vi "Request Data From Flash.vi"() -> (3 "DSM Message":string)   [LabVIEW 2014, in "GEA2_Toolkit.lvlib"]
uses:
  Labview GEA2 Toolkit v2.1/library/GEA2_Toolkit.lvlib
  Custom Pallet Controls/Forward.ctl
panel:
  in  "Number of Bytes (up to 16)":u16
  in  "Starting Index in Record (0-255)":u16
  in  "Record Number (0-Max Record Number)":u16
  out "Description":string="Set Currents"
  in  "Complete":T1
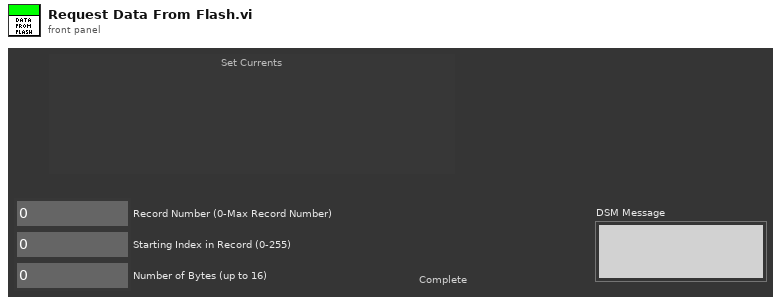
[diagram p1: front panel]
types:
  T1 = typedef "GEA2_Toolkit.lvlib/Forward.ctl" = bool
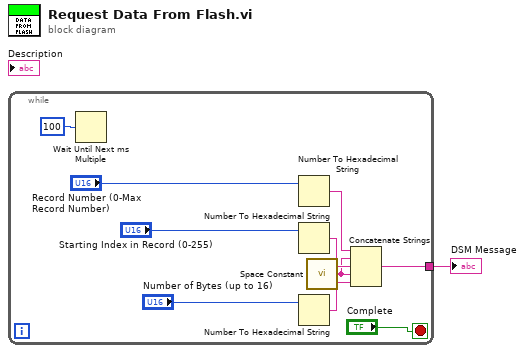
[diagram p0: block diagram]
diagram:
  n1 = while {
    tunnel: [w6] -> w1
    stop <- "Complete" stop-if-true
    n2 = Wait Until Next ms Multiple(millisecond multiple=u32 100) -> ()  [unwired: 1 out]
    n3 = Number To Hexadecimal String(2:"Record Number (0-Max Record Number)") -> (0:w5:string)  [unwired: 1 in]
    n4 = Number To Hexadecimal String(2:"Starting Index in Record (0-255)") -> (0:w4:string)  [unwired: 1 in]
    n5 = Number To Hexadecimal String(2:"Number of Bytes (up to 16)") -> (0:w3:string)  [unwired: 1 in]
    n6 = call <vilib>:"Space Constant.vi"() -> ("String"=w2:string)
    n7 = Concatenate Strings(w5, w2, w4, w2, w3) -> (w6:string)
  }
  "DSM Message" <- w1
